vi "Read Last Result.vi"(11 "Results in":refnum<class "Results.lvclass">) -> (2 "Result":refnum<class "Result.lvclass">, 3 "Results out":refnum<class "Results.lvclass">)   [LabVIEW 2018, in "InfluxDB Client.lvlib" / "Results.lvclass"]
uses:
  Results.lvclass
  Result/Result.lvclass
  Results.lvclass/Results.ctl
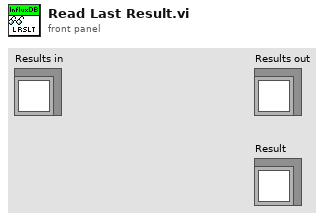
[diagram p1: front panel]
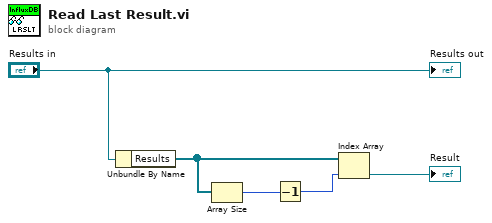
[diagram p0: block diagram]
diagram:
  n1 = Unbundle By Name("Results in") -> ("Results"=w3:refnum<class "Result.lvclass">[])
  n2 = Array Size(array=w3) -> (size(s)=w2:i32)
  n3 = Decrement(x=w2) -> (x-1=w1:i32)
  n4 = Index Array(array=w3, index=w1) -> (element=→"Result":refnum<class "Result.lvclass">)
  "Results out" <- "Results in"
